vi "From Variant.vi"(8 "error in (no error)":errorcluster, 10 "Variant":variant, 11 "Abs_Single Float in":refnum<class "Abs_Single Float.lvclass">) -> (0 "error out":errorcluster, 3 "Abs_Single Float out":refnum<class "Abs_Single Float.lvclass">)   [LabVIEW 2021, in "Abs_Single Float.lvclass"]
uses:
  Abs_Single Float.lvclass
  Support/Type.ctl
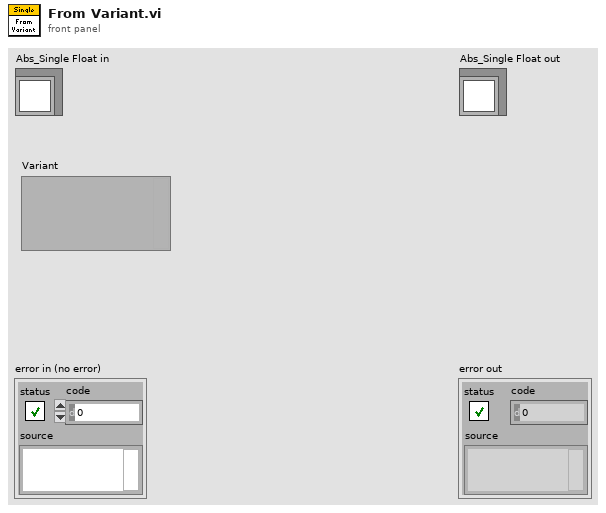
[diagram p1: front panel]
types:
  T1 = typedef "Abs_Single Float.lvclass/Type.ctl" = sgl
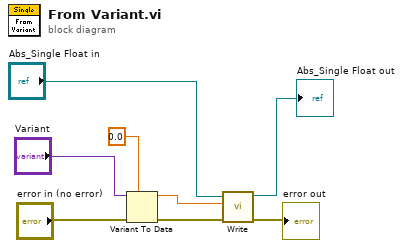
[diagram p0: block diagram]
diagram:
  n1 = Variant To Data(error in="error in (no error)", type=T1 0.0, Variant="Variant") -> (data=w7:T1, error out=w8:errorcluster)
  n2 = call-dynamic "Write.vi"("error in (no error)"=w8, "Value"=w7, "Double Float.lvclass_340760 in"="Abs_Single Float in") -> ("error out"=→"error out":errorcluster, "Double Float.lvclass_340760 out"=→"Abs_Single Float out":refnum<class "Abs_Single Float.lvclass">)  [unwired: 7 in]
